vi "DAQ.setSampling.vi"(8 "error in (no error)":errorcluster, 10 "Sampling":T1={"Sampling"={"Fs"=1000.0, "#s"=128}, "Fs_Out"=204789.0} {"Sampling"."Fs" format="%#_13g"}, 11 "Instrument.DAQ":refnum<class "Instrument.DAQ.lvclass">) -> (0 "error out":errorcluster, 3 "Instrument.DAQ out":refnum<class "Instrument.DAQ.lvclass">)   [LabVIEW 2019, in "Instrument.Lockin.lvlib" / "Instrument.DAQ.lvclass"]
doc: "---------------------------------------------------------------\nJKI State Machine Objects™\nhttp://jki.net/state-machine-objects/\nCopyright (C) 2005-2015, JKI <info@jki.net>\nALL RIGHTS RESERVEDJKI State Machine Objects (SMO) 1.0.0.4\nJKI - JKI\nCopyright (c) 2015, JKI"
uses:
  Instrument.DAQ.lvclass
  Typedefs/DAQ.Sampling--Cluster.ctl
  Typedefs/DAQ.Sampling.Sampling--Cluster.ctl
  Typedefs/PrivateEvents--DAQ.setSampling.ctl
  Instrument.DAQ.lvclass/Instrument.DAQ.ctl
panel:
  # "For instructions on how to use the JKI State Machine Objects, examples and video tutorials, visit:\nhttp://jki.net/state-machine-objects/\n\nJKI State Machine Objects™\nhttp://jki.net/state-machine-objects/\nCopyright (C) 2005-2015, JKI <info@jki.net>\nALL RIGHTS RESERVED"
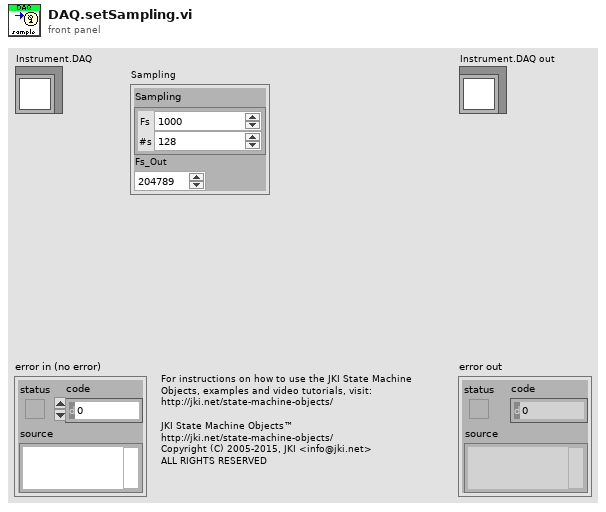
[diagram p1: front panel]
types:
  T1 = typedef "Instrument.Lockin.lvlib/Instrument.DAQ.lvclass/DAQ.Sampling--Cluster.ctl" = cluster{"Sampling":T2, "Fs_Out":dbl}
  T2 = typedef "Instrument.Lockin.lvlib/Instrument.DAQ.lvclass/DAQ.Sampling.Sampling--Cluster.ctl" = cluster{"Fs":dbl, "#s":i32}
  T3 = typedef "Instrument.Lockin.lvlib/Instrument.DAQ.lvclass/PrivateEvents--DAQ.setSampling.ctl" = cluster{"Sampling":T1}
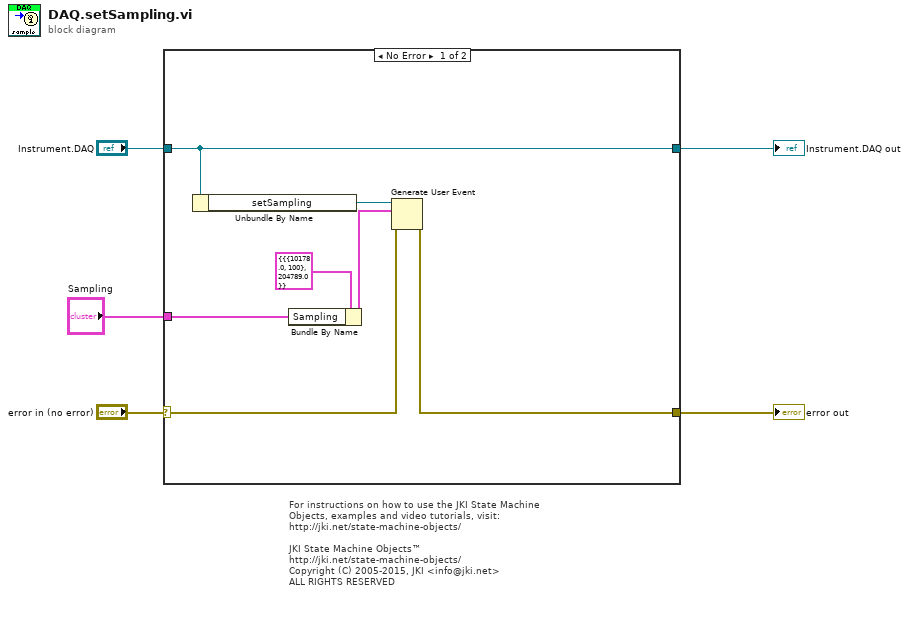
[diagram p0: block diagram]
diagram:
  # "For instructions on how to use the JKI State Machine Objects, examples and video tutorials, visit:\nhttp://jki.net/state-machine-objects/\n\nJKI State Machine Objects™\nhttp://jki.net/state-machine-objects/\nCopyright (C) 2005-2015, JKI <info@jki.net>\nALL RIGHTS RESERVED"
  n1 = case shown="No Error" "error in (no error)" {
    selector: "error in (no error)" -> [w12 w14]
    tunnel: [w10 w14] -> w4
    tunnel: [w9 w13] -> w5
    tunnel: "Instrument.DAQ" -> [w9 w13]
    tunnel: "Sampling" -> [w7 _]
    frame No Error {
      n2 = Unbundle By Name(w9) -> ("setSampling"=w11:refnum<user-event>)
      n3 = Bundle By Name(cluster=T3 {"Sampling"={"Sampling"={"Fs"=10178.0, "#s"=100}, "Fs_Out"=204789.0}} ("setSampling"), "Sampling"=w7) -> (w6:T3)
      n4 = Generate User Event(user event=w11, event data cluster=w6, error in=w12) -> (error out=w10:errorcluster)  [unwired: 1 in, 1 out]
    }
    frame Error {
    }
  }
  "error out" <- w4
  "Instrument.DAQ out" <- w5
